vi "Remove Test Channel.vi"(8 "error in (no error)":errorcluster, 11 "Test Channel Model in":refnum<class "Test Channel Model.lvclass">) -> (0 "error out":errorcluster, 3 "Test Channel Model out":refnum<class "Test Channel Model.lvclass">)   [LabVIEW 2013, in "Test Channel Model.lvlib" / "Test Channel Model.lvclass"]
uses:
  Test Channel Model.lvclass
  Test Channel Model.lvclass/Test Channel Model.ctl
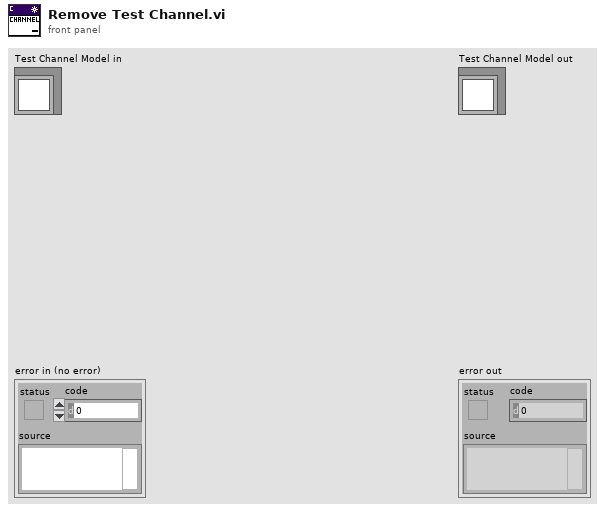
[diagram p1: front panel]
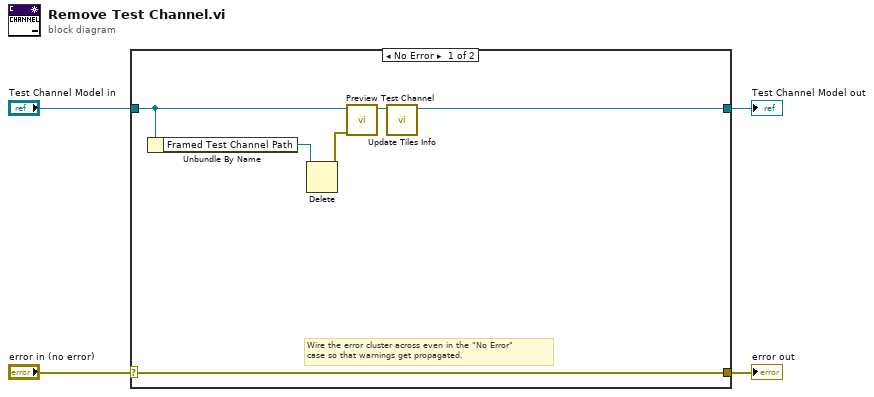
[diagram p0: block diagram]
diagram:
  n1 = case shown="No Error" "error in (no error)" {
    selector: "error in (no error)" -> [w10 w12]
    tunnel: [w10 w12] -> w3
    tunnel: [w5 w11] -> w1
    tunnel: "Test Channel Model in" -> [w6 w11]
    frame No Error {
      # "Wire the error cluster across even in the \"No Error\"\ncase so that warnings get propagated."
      n2 = Unbundle By Name(w6) -> ("Framed Test Channel Path"=w8:path)
      n3 = Delete(path (use dialog)=w8) -> (error out=w7:errorcluster)  [unwired: 4 in, 2 out]
      n4 = call "Preview Test Channel.vi"("error in (no error)"=w7, "Test Channel Model in"=w6) -> ("Test Channel Model out"=w9:refnum<class "Test Channel Model.lvclass">)  [unwired: 8 in, 1 out]
      n5 = call "Update Tiles Info.vi"("Test Channel Model in"=w9) -> ("Test Channel Model out"=w5:refnum<class "Test Channel Model.lvclass">)  [unwired: 9 in, 1 out]
    }
    frame Error {
    }
  }
  "error out" <- w3
  "Test Channel Model out" <- w1
